vi "loadHTSocketLog.vi"(11 "file (use dialog)":path=path "C:/temp/ht/Socket/SocketLog.txt") -> ()   [LabVIEW 2012]
uses:
  <vilib>/addons/database/Connection.llb/DB Tools Open Connec (Path).vi
  <vilib>/addons/database/Connection.llb/Conn Execute.vi
  <vilib>/addons/database/Recordset.llb/Rec Destroy - Connection.vi
  <vilib>/addons/database/NI_Database_API.lvlib
panel:
  out "concatenated string":string
  out "after substring":string
  out "date/time string":string
  out "text":string
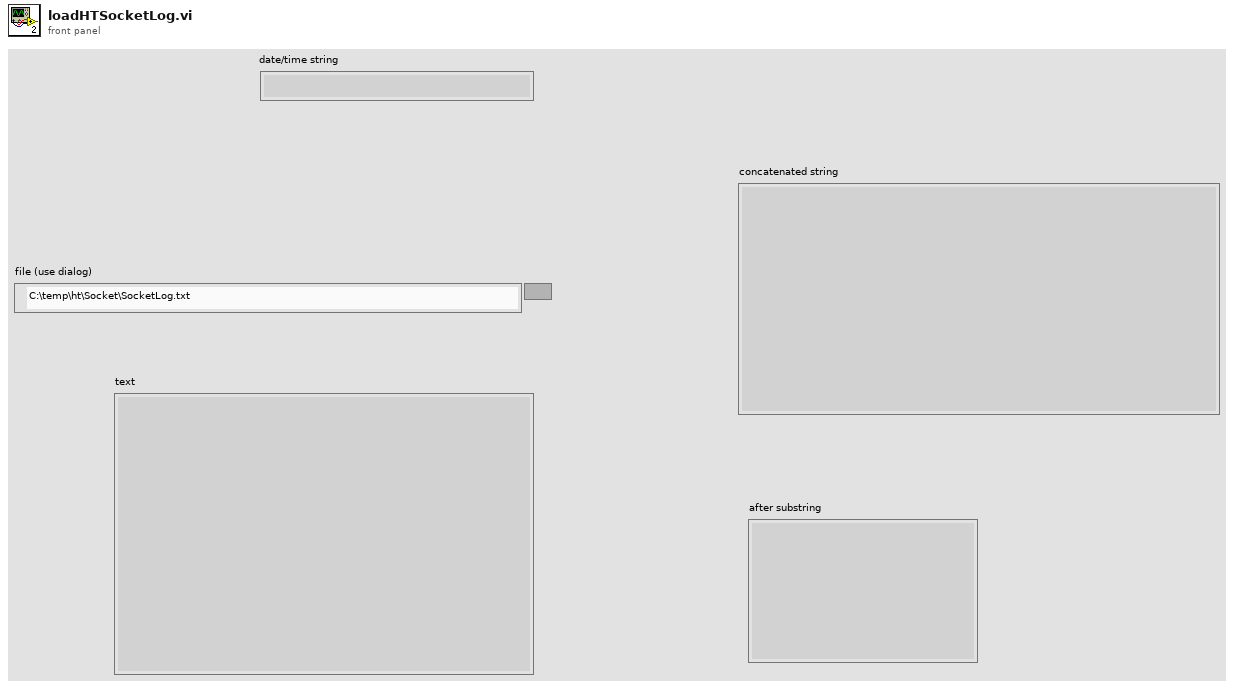
[diagram p1: front panel]
types:
  T1 = typedef "NI_Database_API.lvlib/Conn ObjectReference.ctl" = refnum<k1>
  T2 = typedef "NI_Database_API.lvlib/Rec ObjectReference.ctl" = refnum<k1>
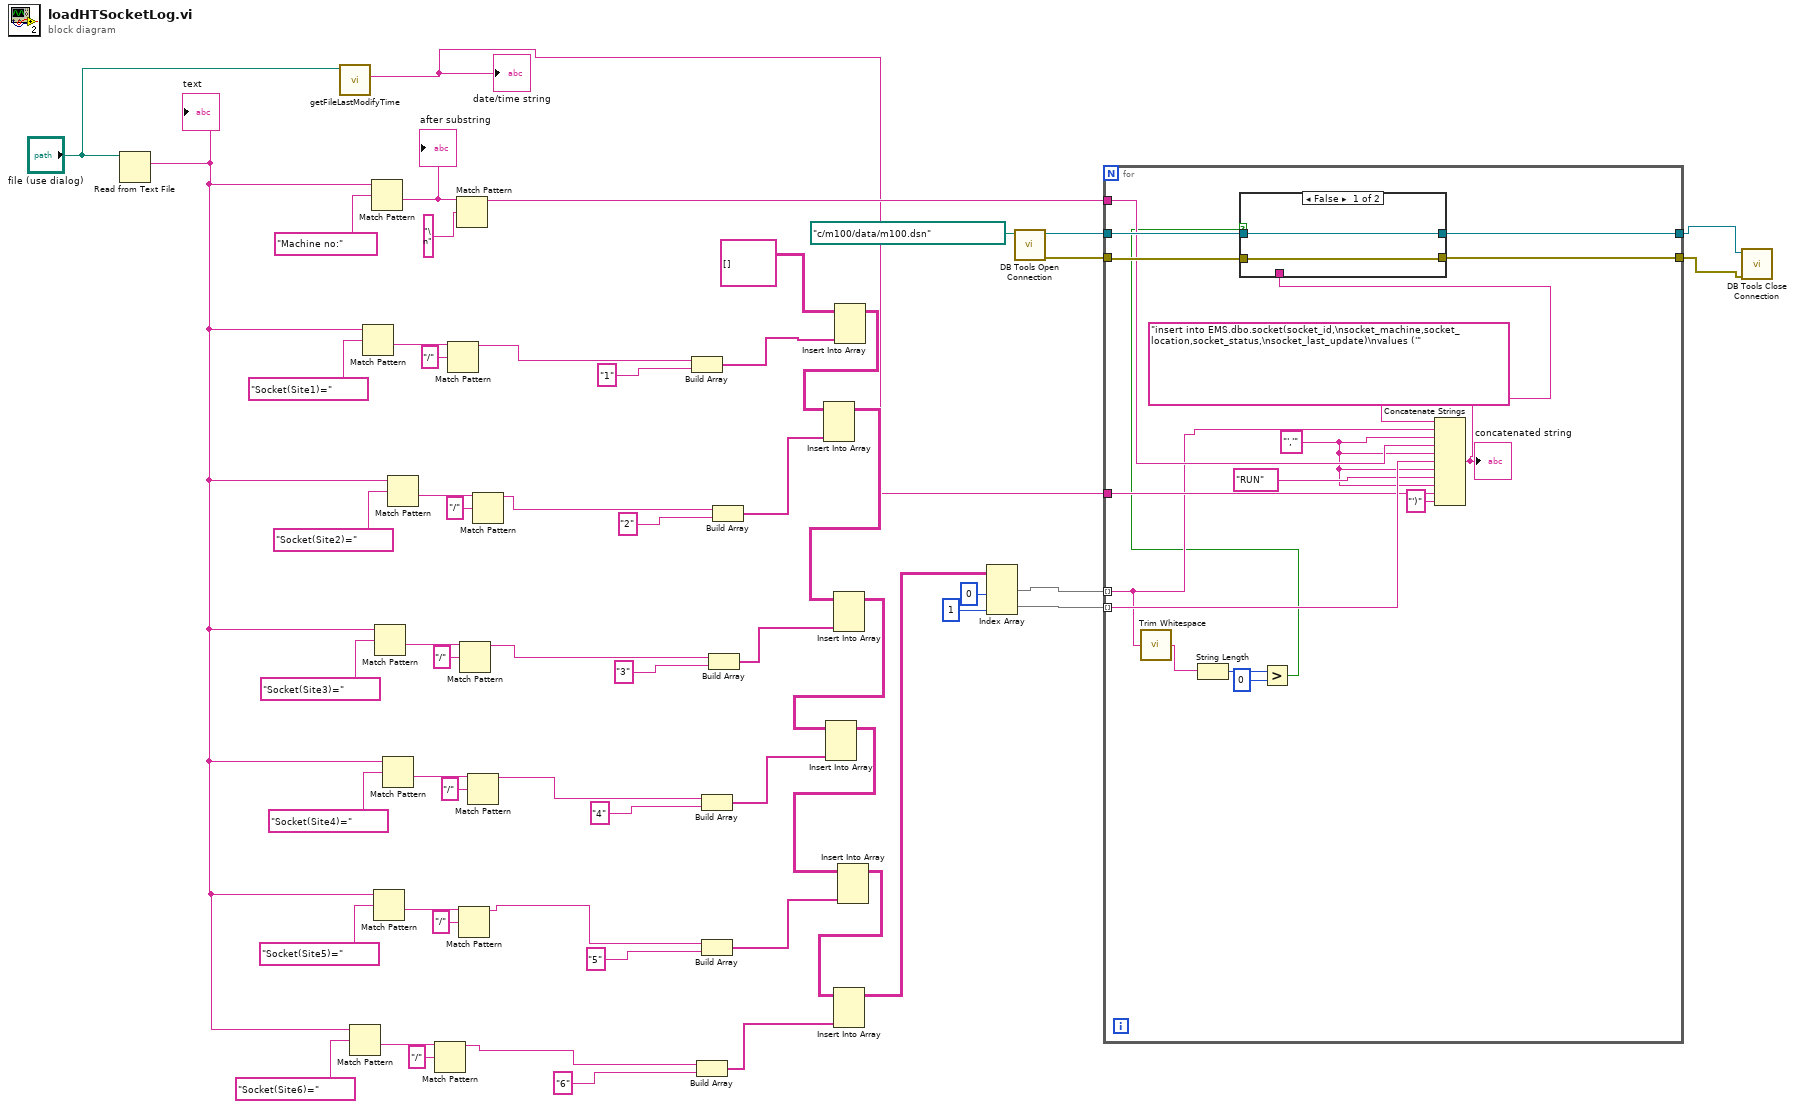
[diagram p0: block diagram]
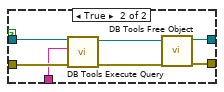
[diagram p2: hidden frame]
diagram:
  n1 = Read from Text File(file (use dialog)="file (use dialog)") -> (text=w38:string)  [unwired: 3 in, 3 out]
  "text" <- w38
  n2 = call "getFileLastModifyTime.vi"("path"="file (use dialog)") -> ("date/time string"=w3:string)  [unwired: 10 in]
  "date/time string" <- w3
  n3 = Match Pattern(string=w38, regular expression="Socket(Site6)=") -> (after substring=w40:string)  [unwired: 1 in, 3 out]
  n4 = Match Pattern(string=w38, regular expression="Socket(Site1)=") -> (after substring=w55:string)  [unwired: 1 in, 3 out]
  n5 = Match Pattern(string=w38, regular expression="Machine no:") -> (after substring=w58:string)  [unwired: 1 in, 3 out]
  "after substring" <- w58
  n6 = Match Pattern(string=w38, regular expression="Socket(Site5)=") -> (after substring=w43:string)  [unwired: 1 in, 3 out]
  n7 = Match Pattern(string=w38, regular expression="Socket(Site3)=") -> (after substring=w49:string)  [unwired: 1 in, 3 out]
  n8 = Match Pattern(string=w38, regular expression="Socket(Site4)=") -> (after substring=w46:string)  [unwired: 1 in, 3 out]
  n9 = Match Pattern(string=w38, regular expression="Socket(Site2)=") -> (after substring=w52:string)  [unwired: 1 in, 3 out]
  n10 = Match Pattern(string=w40, regular expression="/") -> (before substring=w28:string)  [unwired: 1 in, 3 out]
  n11 = Match Pattern(string=w55, regular expression="/") -> (before substring=w36:string)  [unwired: 1 in, 3 out]
  n12 = Match Pattern(string=w58, regular expression="\n") -> (before substring=w4:string)  [unwired: 1 in, 3 out]
  n13 = Match Pattern(string=w43, regular expression="/") -> (before substring=w27:string)  [unwired: 1 in, 3 out]
  n14 = Match Pattern(string=w49, regular expression="/") -> (before substring=w32:string)  [unwired: 1 in, 3 out]
  n15 = Match Pattern(string=w46, regular expression="/") -> (before substring=w26:string)  [unwired: 1 in, 3 out]
  n16 = Match Pattern(string=w52, regular expression="/") -> (before substring=w34:string)  [unwired: 1 in, 3 out]
  n17 = Build Array(w36, "1" ("element")) -> (w16:string[])
  n18 = Build Array(w28, "6" ("element")) -> (w17:string[])
  n19 = Build Array(w26, "4" ("element")) -> (w21:string[])
  n20 = Build Array(w27, "5" ("element")) -> (w19:string[])
  n21 = Build Array(w32, "3" ("element")) -> (w23:string[])
  n22 = Build Array(w34, "2" ("element")) -> (w25:string[])
  n23 = Insert Into Array(array=string[][] [], new element=w16) -> (w15:string[][])  [unwired: 2 in]
  n24 = Insert Into Array(array=w15, new element=w25) -> (w24:string[][])  [unwired: 2 in]
  n25 = Insert Into Array(array=w24, new element=w23) -> (w22:string[][])  [unwired: 2 in]
  n26 = Insert Into Array(array=w22, new element=w21) -> (w20:string[][])  [unwired: 2 in]
  n27 = Insert Into Array(array=w20, new element=w19) -> (w18:string[][])  [unwired: 2 in]
  n28 = Insert Into Array(array=w18, new element=w17) -> (w13:string[][])  [unwired: 2 in]
  n29 = Index Array(array=w13, index (col) #1=0 ("disabled index (col)"), index (col) #2=1 ("index (col)")) -> (element #1=w1:string[], element #2=w12:string[])  [unwired: 2 in]
  n30 = call-poly <vilib>:"DB Tools Open Connection.vi"("connection information"=path "c:/m100/data/m100.dsn") -> ("error out"=w6:errorcluster, "connection reference"=w8:T1)  [unwired: 7 in]
  n31 = for {
    tunnel: w1 -> [w62] mode=indexing
    tunnel: w12 -> [w70] mode=indexing
    tunnel: w8 -> [w76]
    tunnel: [w75] -> w7
    tunnel: w6 -> [w73]
    tunnel: [w74] -> w5
    tunnel: w4 -> [w71]
    tunnel: w3 -> [w67]
    w68 = "','" ("string")
    n32 = call <vilib>:"Trim Whitespace.vi"("string"=w62) -> ("trimmed string"=w61:string)  [unwired: 1 in]
    n33 = String Length(string=w61) -> (length=w64:i32)
    n34 = Greater?(x=w64, y=0) -> (0:w60:bool)
    n35 = Concatenate Strings("insert into EMS.dbo.socket(socket_id,\nsocket_machine,socket_location,socket_status,\nsocket_last_update)\nvalues ('" ("string"), w62, w68, w71, w68, w70, w68, "RUN" ("string"), w68, w67, "')" ("string")) -> (w65:string)
    "concatenated string" <- w65
    n36 = case shown="False" w60 {
      tunnel: w76 -> [w78 w85]
      tunnel: [w78 w83] -> w75
      tunnel: [w77 w81] -> w74
      tunnel: w73 -> [w77 w80]
      tunnel: w65 -> [_ w79]
      frame False {
      }
      frame True {
        n37 = call-poly <vilib>:"DB Tools Execute Query.vi"("error in (no error)"=w80, "SQL query"=w79, "connection reference"=w85) -> ("error out"=w82:errorcluster, "recordset reference"=w84:T2)  [unwired: 5 in]
        n38 = call-poly <vilib>:"DB Tools Free Object.vi"("error in (no error)"=w82, "recordset reference"=w84) -> ("error out"=w81:errorcluster, "connection reference"=w83:T1)  [unwired: 8 in]
      }
    }
  }
  n39 = call <vilib>:"DB Tools Close Connection.vi"("error in (no error)"=w5, "connection reference"=w7) -> ()  [unwired: 5 in, 1 out]
